vi "Simple Cycle.vi"(8 "Error In":errorcluster, 10 "Cycle settings":T1, 11 "VISA in":refnum<visa-resource-name>) -> (0 "Error Out":errorcluster, 3 "VISA out":refnum<visa-resource-name>)   [LabVIEW 2014]
uses:
  LV Library/Typedef/Move type.ctl
  LV Library/Motor manager.lvlib
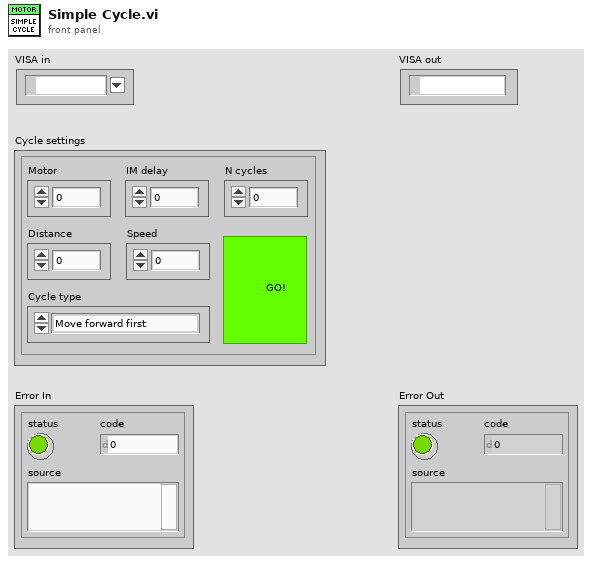
[diagram p1: front panel]
types:
  T1 = cluster{"Motor":u8, "Distance":i32, "Speed":sgl, "IM delay":i32, "Cycle type":enum16{"Move forward first", "Move backward first"}, "N cycles":i32, "Go cycle":bool}
  T2 = typedef "Motor manager.lvlib/Move type.ctl" = enum16{"Move forward", "Move backward", "Cycle (forward first)", "Cycle (backward first)", "Move step forward", "Move step backward"}
  T3 = enum16{"Move forward first", "Move backward first"}
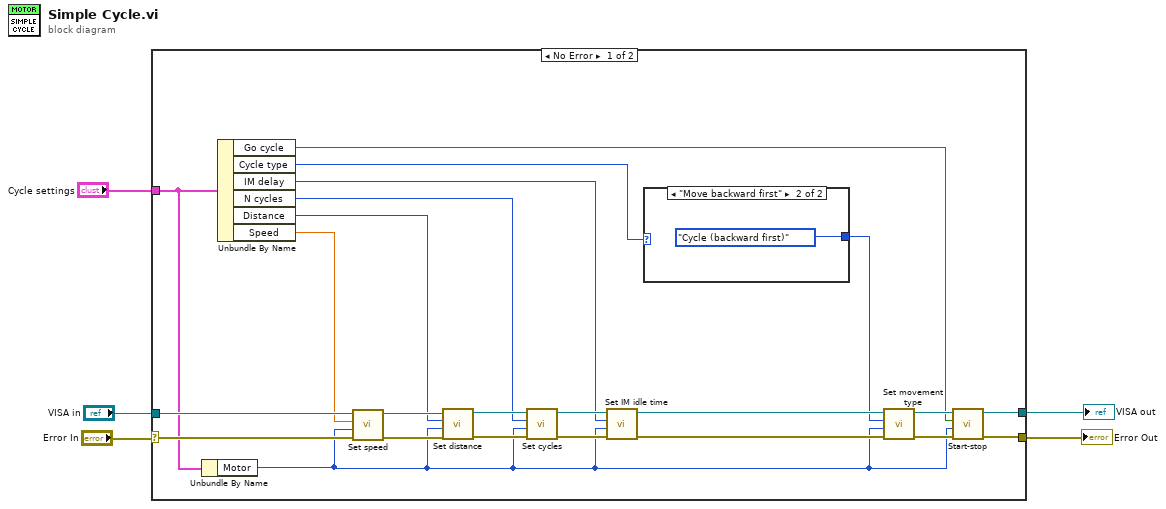
[diagram p0: block diagram]
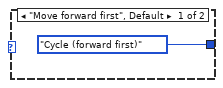
[diagram p2: hidden frame]
diagram:
  n1 = case shown="No Error" "Error In" {
    selector: "Error In" -> [w28 w31]
    tunnel: [w12 w31] -> w4
    tunnel: "Cycle settings" -> [w20 _]
    tunnel: "VISA in" -> [w24 w32]
    tunnel: [w11 w32] -> w1
    frame No Error {
      n2 = Unbundle By Name(w20) -> ("Motor"=w9:u8)
      n3 = Unbundle By Name(w20) -> ("Go cycle"=w6:bool, "Cycle type"=w8:T3, "IM delay"=w16:i32, "N cycles"=w17:i32, "Distance"=w18:i32, "Speed"=w19:sgl)
      n4 = call "Set speed.vi"("Error In"=w28, "Motor index"=w9, "Speed"=w19, "VISA resource in"=w24) -> ("Error Out"=w27:errorcluster, "VISA resource out"=w23:refnum<visa-resource-name>)  [unwired: 6 in]
      n5 = call "Set distance.vi"("Error In"=w27, "Motor index"=w9, "Travel distance"=w18, "VISA resource in"=w23) -> ("Error Out"=w26:errorcluster, "VISA resource out"=w22:refnum<visa-resource-name>)  [unwired: 6 in]
      n6 = call "Set cycles.vi"("Error In"=w26, "Motor index"=w9, "N cycles"=w17, "VISA resource in"=w22) -> ("Error Out"=w25:errorcluster, "VISA resource out"=w21:refnum<visa-resource-name>)  [unwired: 6 in]
      n7 = call "Set IM idle time.vi"("Error In"=w25, "Motor index"=w9, "IM Idle time"=w16, "VISA resource in"=w21) -> ("Error Out"=w14:errorcluster, "VISA resource out"=w15:refnum<visa-resource-name>)  [unwired: 6 in]
      n8 = case shown="\"Move backward first\"" w8 {
        tunnel: [Move_type."Cycle (forward first)" ("Movement type") Move_type."Cycle (backward first)" ("Movement type")] -> w7
        frame "Move forward first", Default {
        }
        frame "Move backward first" {
        }
      }
      n9 = call "Set movement type.vi"("Error In"=w14, "Motor index"=w9, "Movement type"=w7, "VISA resource in"=w15) -> ("Error Out"=w13:errorcluster, "VISA resource out"=w10:refnum<visa-resource-name>)  [unwired: 6 in]
      n10 = call "Start-stop.vi"("Error In"=w13, "Motor index"=w9, "Go"=w6, "VISA resource in"=w10) -> ("Error Out"=w12:errorcluster, "VISA resource out"=w11:refnum<visa-resource-name>)  [unwired: 6 in]
    }
    frame Error {
    }
  }
  "VISA out" <- w1
  "Error Out" <- w4
